vi "TCL Get Message.vi"() -> (0 "Text":string, 1 "TCL Message Type":T1(ring)=enum."Address=")   [LabVIEW 2009]
panel:
  in  "Timeout ms (-1)":i32=-1
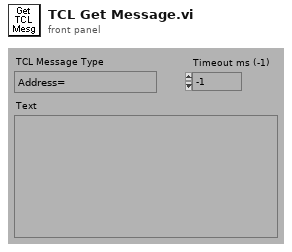
[diagram p1: front panel]
types:
  T1 = enum16{"No Message", "Bad Message", "NewEventFile", "NewBaseFile", "Event=", "Ping=", "Address=", "Stop"}
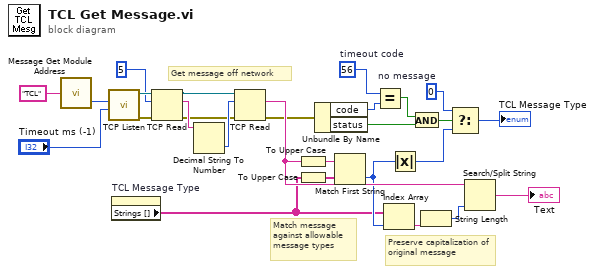
[diagram p0: block diagram]
diagram:
  w7 = 0  # no message
  w10 = 56  # timeout code
  # "Get message off network"
  # "Match message against allowable message types"
  # "Preserve capitalization of original message"
  n1 = call "Message Get Module Address.vi"("Module"="TCL") -> ("Port"=w4:u16)  [unwired: 1 out]
  n2 = call <vilib>:"TCP Listen.vi"("timeout ms (wait forever: -1)"="Timeout ms (-1)", "port"=w4) -> ("error out"=w22:errorcluster, "connection ID"=w23:refnum<k5>)  [unwired: 6 in, 2 out]
  n3 = property on="TCL Message Type" class="Enum (strict)"() -> ("Strings []"=w3:string[])  [unwired: 2 in, 2 out]
  n4 = TCP Read(connection ID=w23, bytes to read=5 ("size of message length"), error in (no error)=w22) -> (connection ID out=w18:refnum<k5>, data out=w20:string, error out=w17:errorcluster)  [unwired: 2 in]
  n5 = Decimal String To Number(string=w20) -> (number=w19:i32)  [unwired: 2 in, 1 out]
  n6 = TCP Read(connection ID=w18, bytes to read=w19, error in (no error)=w17) -> (data out=w16:string, error out=w14:errorcluster)  [unwired: 2 in, 1 out]
  n7 = To Upper Case(1:w16) -> (0:w27:string)
  n8 = To Upper Case(1:w3) -> (0:w26:string[])
  n9 = Unbundle By Name(w14) -> ("code"=w11:i32, "status"=w13:bool)
  n10 = Match First String(2:w26, 3:w27) -> (0:w9:i32)  [unwired: 1 out]
  n11 = Equal?(x=w10, y=w11) -> (x = y?=w12:bool)
  n12 = Index Array(array=w3, index=w9) -> (element=w24:string)
  n13 = Absolute Value(x=w9) -> (abs(x)=w6:i32)
  n14 = And(x=w12, y=w13) -> (x .and. y?=w8:bool)
  n15 = String Length(string=w24) -> (length=w25:i32)
  n16 = Select(t=w7, s=w8, f=w6) -> (s? t:f=→"TCL Message Type":i32)
  n17 = Search/Split String(string=w16, offset (0)=w25) -> (match + rest of string=→"Text":string)  [unwired: 1 in, 2 out]
